vi "IsData.vi"(1 "File":path=path "E:/Programs/AWG/200 MHz.txt") -> (0 "True/False":bool)   [LabVIEW 2014]
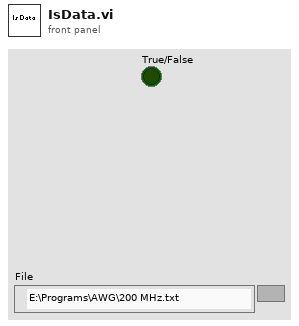
[diagram p1: front panel]
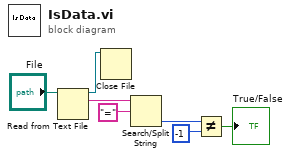
[diagram p0: block diagram]
diagram:
  n1 = Read from Text File(file (use dialog)="File") -> (refnum out=w1:refnum<file>, text=w6:string)  [unwired: 3 in, 2 out]
  n2 = Close File(refnum=w1) -> ()  [unwired: 1 in, 2 out]
  n3 = Search/Split String(string=w6, search string/char (-)="=") -> (offset of match=w5:i32)  [unwired: 1 in, 2 out]
  n4 = Not Equal?(x=w5, y=-1) -> (x != y?=→"True/False":bool)
